vi "main.vi"() -> ()   [LabVIEW 2026]
panel:
  out "System Status":string
  in  "Stop":bool
  in  "RUN":bool
  out "PASS / FAIL":bool
  out "Sensor Data Waveform":dbl(graph)
  out "Voltage (V)":dbl(knob) scale=0.0..10.0
  out "Humidity (%)":dbl(knob) scale=0.0..10.0
  out "Thermometer('c)":dbl(slide) scale=0.0..100.0
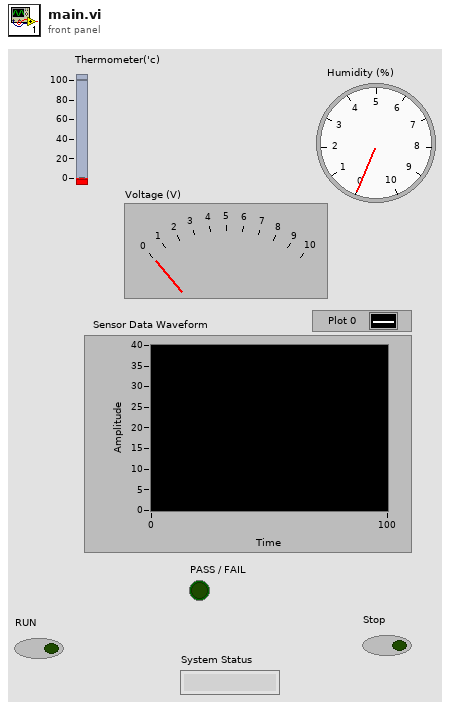
[diagram p1: front panel]
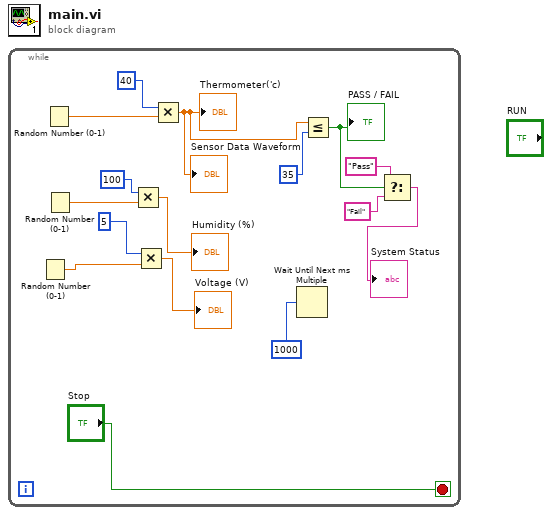
[diagram p0: block diagram]
diagram:
  n1 = while {
    stop <- "Stop" stop-if-true
    n2 = Random Number (0-1)() -> (number: 0 to 1=w9:dbl)
    n3 = Random Number (0-1)() -> (number: 0 to 1=w15:dbl)
    n4 = Random Number (0-1)() -> (number: 0 to 1=w13:dbl)
    n5 = Multiply(x=100, y=w13) -> (x*y=→"Humidity (%)":dbl)
    n6 = Multiply(x=5, y=w9) -> (x*y=→"Voltage (V)":dbl)
    n7 = Multiply(x=40, y=w15) -> (x*y=w1:dbl)
    "Thermometer('c)" <- w1
    "Sensor Data Waveform" <- w1
    n8 = Wait Until Next ms Multiple(millisecond multiple=u32 1000) -> ()  [unwired: 1 out]
    n9 = Less Or Equal?(x=w1, y=35) -> (x <= y?=w5:bool)
    "PASS / FAIL" <- w5
    n10 = Select(t="Pass", s=w5, f="Fail") -> (s? t:f=→"System Status":string)
  }
